vi "Load Waveform List from File.vi"(8 "error in (no error)":errorcluster) -> (0 "error out":errorcluster, 2 "Original Waveforms":waveform(dbl)[](array[waveform]), 3 "Waveform Loaded?":bool)   [LabVIEW 2021]
uses:
  <vilib>/ErrorRing/Error Ring.xnode
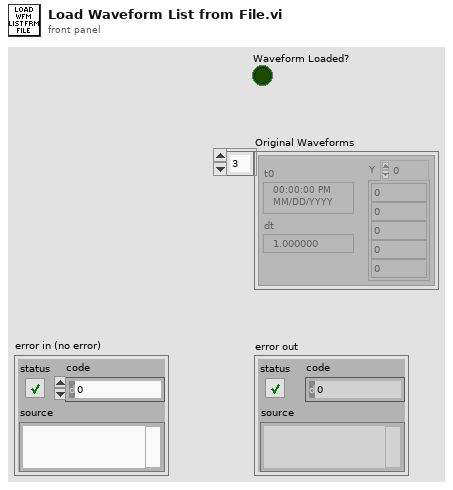
[diagram p1: front panel]
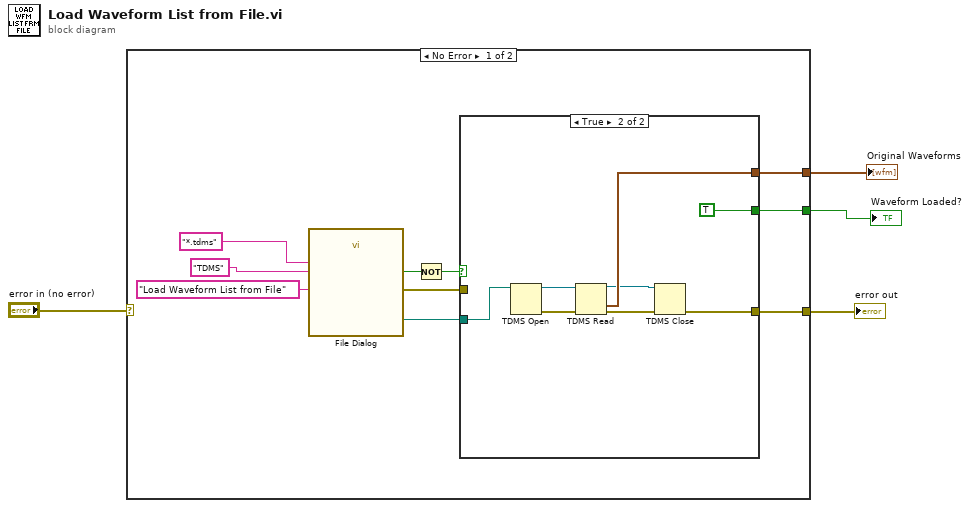
[diagram p0: block diagram]
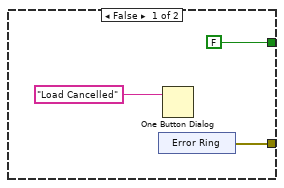
[diagram p2: hidden frame]
diagram:
  n1 = case shown="No Error" "error in (no error)" {
    selector: "error in (no error)" -> [_ w27]
    tunnel: [w7 w27] -> w4
    tunnel: [w6 _] -> w2
    tunnel: [w5 _] -> w1
    frame No Error {
      n2 = call "File Dialog"("prompt"="Load Waveform List from File", "pattern (all files)"="*.tdms" ("prompt"), "pattern label"="TDMS" ("prompt")) -> ("selected path"=w11:path, "cancelled"=w10:bool, "error out"=w8:errorcluster)  [unwired: 9 in, 1 out]
      n3 = Not(x=w10) -> (.not. x?=w9:bool)
      n4 = case shown="True" w9 {
        tunnel: w11 -> [_ w24]
        tunnel: w8 -> [_ _]
        tunnel: [w16 w20] -> w7
        tunnel: [_ w26] -> w6
        tunnel: [FALSE TRUE] -> w5
        frame False {
          n5 = xnode "Error Ring"() -> ("error out"=w16:errorcluster)
          n6 = One Button Dialog(message="Load Cancelled") -> ()  [unwired: 1 in, 1 out]
        }
        frame True {
          n7 = TDMS Open(11:w24) -> (0:w23:errorcluster, 3:w19:refnum<k34>)  [unwired: 6 in]
          n8 = TDMS Read(0:w19, 11:w23) -> (4:w21:refnum<k34>, 10:w26:waveform(dbl)[], 15:w22:errorcluster)  [unwired: 6 in, 3 out]
          n9 = TDMS Close(8:w22, 11:w21) -> (0:w20:errorcluster)  [unwired: 1 out]
        }
      }
    }
    frame Error {
    }
  }
  "error out" <- w4
  "Original Waveforms" <- w2
  "Waveform Loaded?" <- w1
